vi "Emballage affiche cmde non terminée_V2.vi"(6 "error in (no error)":errorcluster caption="entrée d'erreur (pas d'erreur)", 11 "N° cmde en cours":string(combo)="02302/08-01.07.01", 16 "melange des lots possibles ?":bool=TRUE) -> (12 "DATA cmde":T1={"n°article FAS"="", "n° cmde FAS"="02302/08-01.07.01", "quantité cmde"="100", "ID LIG cmde"="225785", "n° cmde client"="120189 / 109644     ", "nom client"="Fluid Automat. Systems GmbH", "n° article client"="20869", "indice revision client"="03    ", "société de facturation"="FAS Medic SA                            ", "langue a utiliser"="ALL"}, 14 "Nombre de carton complets":i16=2, 15 "Nombre de carton+1 :":i16=2, 17 "pièce(s)":i16=8, 18 "#valve déjà emballée":i32, 19 "Commencer Une autre commande OUT":bool, 20 "Recommencer la commande OUT":bool, 21 "No commande FAS":string, 22 "Pb lecture cmde":bool, 23 "Continuer l'emballage  OUT":bool=TRUE, 24 "Quantité de la commande":string="4", 25 "Commande interne":bool, 26 "error out":errorcluster caption="sortie d'erreur")   [LabVIEW 2020]
uses:
  Modules/FS/60_FS_Controles/60_FS_SetGet.ctl
panel:
  out "temps [s]":dbl
  out "cmd non fini":string[](array[string])
  in  "Commencer Une autre commande":bool
  in  "Recommencer la commande":bool
  in  "Continuer l'emballage":bool
  # "Commande n°\n\nnon terminée !"
  # "Nombre de cartons emballés :"
  # "Vous avez \n dans le carton n°"
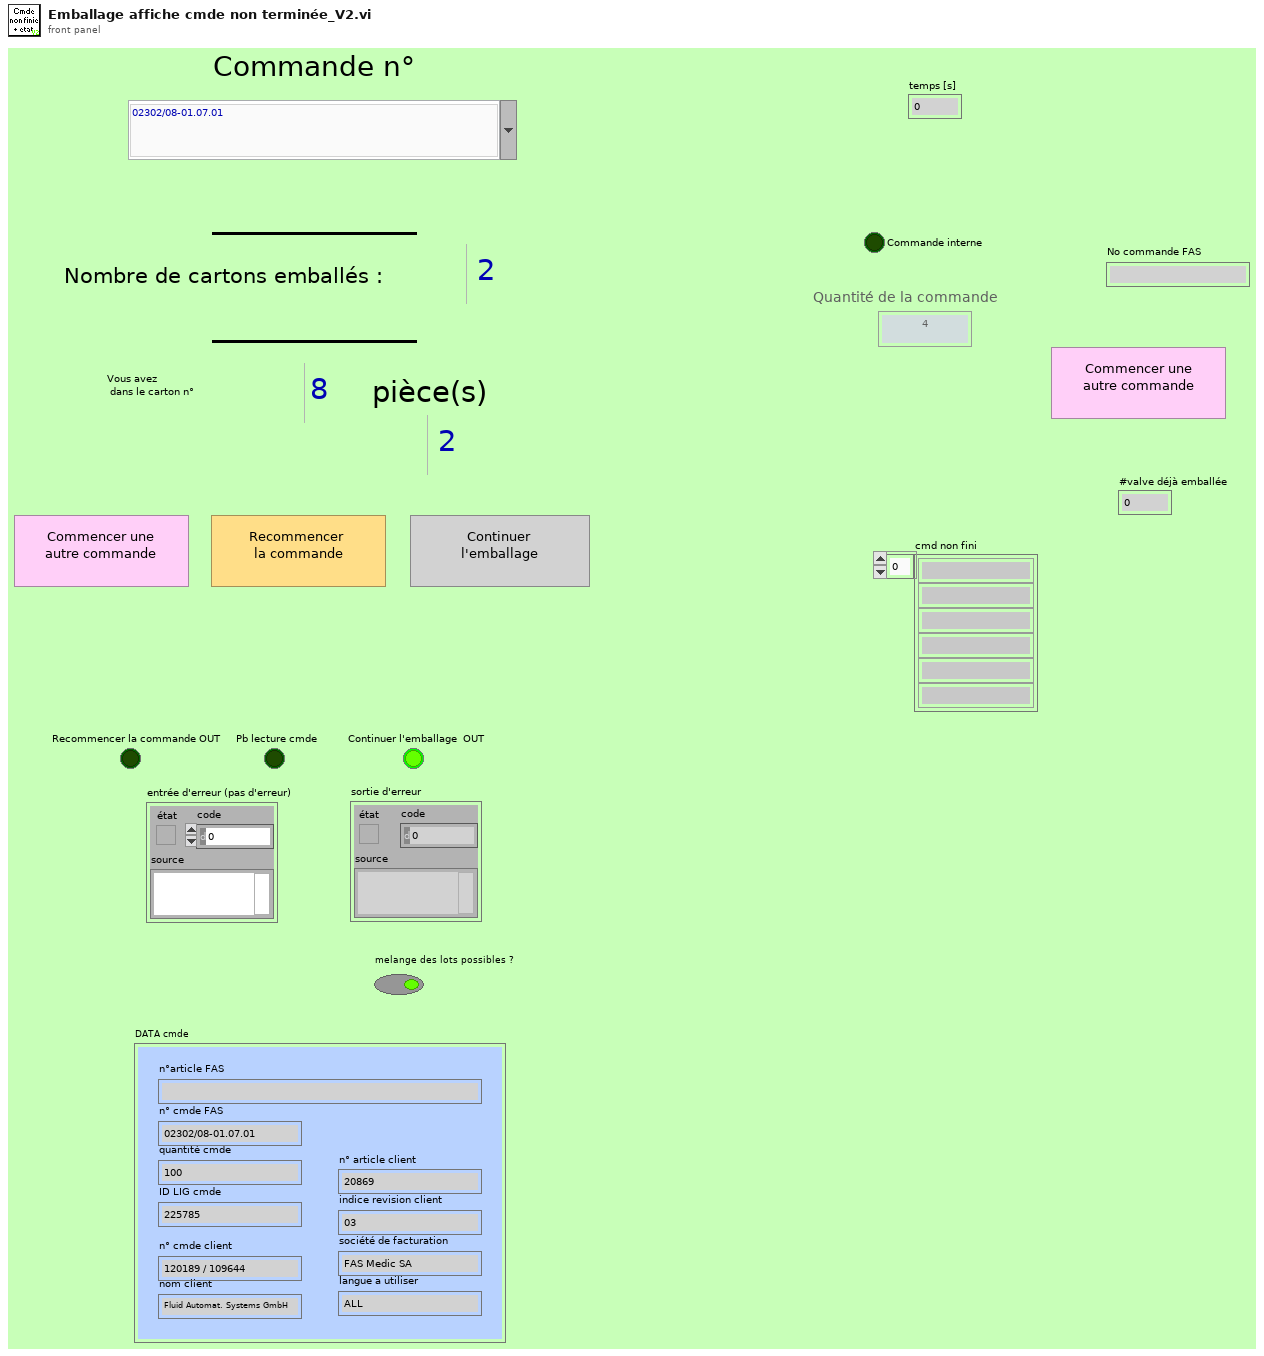
[diagram p1: front panel]
types:
  T1 = typedef "DATA commande.ctl" = cluster{"n°article FAS":string, "n° cmde FAS":string, "quantité cmde":string, "ID LIG cmde":string, "n° cmde client":string, "nom client":string, "n° article client":string, "indice revision client":string, "société de facturation":string, "langue a utiliser":string}
  T2 = enum8{"Enabled", "Disabled", "Disabled and Grayed Out"}
  T3 = typedef "60_FS_SetGet.ctl" = enum16{"set", "get"}
  T4 = typedef "Emballage_BDD_param_Produit.ctl" = cluster{"No_Valve_FAS":string, "suffixe":string, "designation":string, "indice_produit":string, "code_barre_fixe":string, "affiche_code_barre_client":string, "affiche_no_client":string, "Nb_vlve_par_carton":u16, "melange_des_lots_possible":string, "id_article":string, "Indice_Rev":string, "Famille":string, "date":string, "code_barre_fixe_Fin":string, "Longeur_No_Serie":string}
  T5 = typedef "60_FS_CLT_Chemins.ctl" = cluster{"Racine_local":path, "Racine_reseau":path, "Racine_Support_Application":path, "Fichier_Journalisation":path, "Connexion_BDD_VSX":path, "Connexion_BDD_PLZ":path}
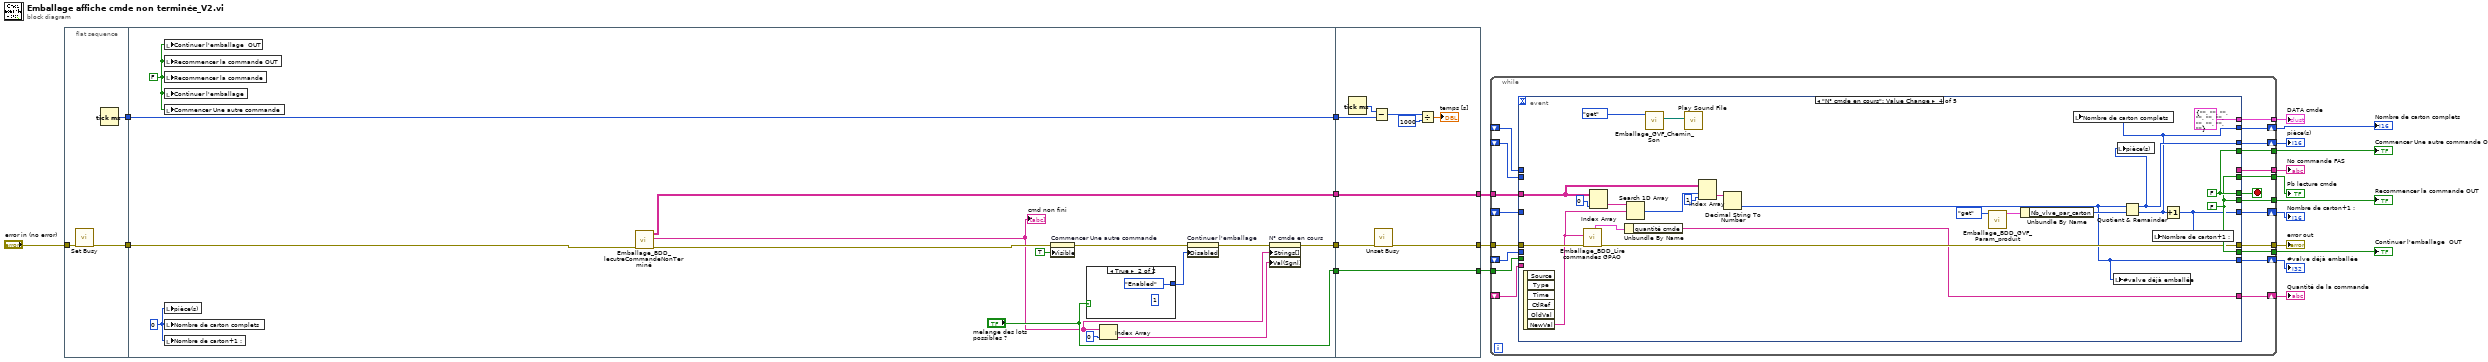
[diagram p0: block diagram]
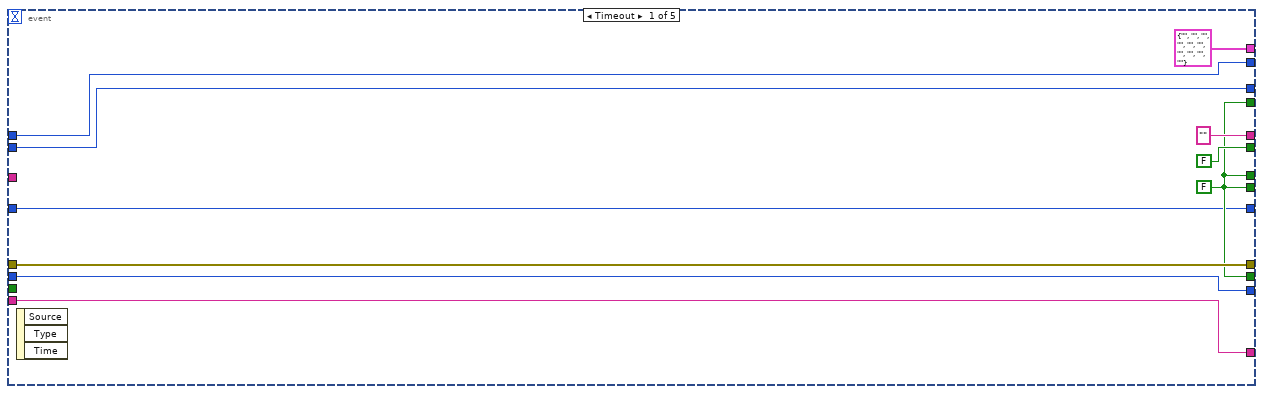
[diagram p2: hidden frame]
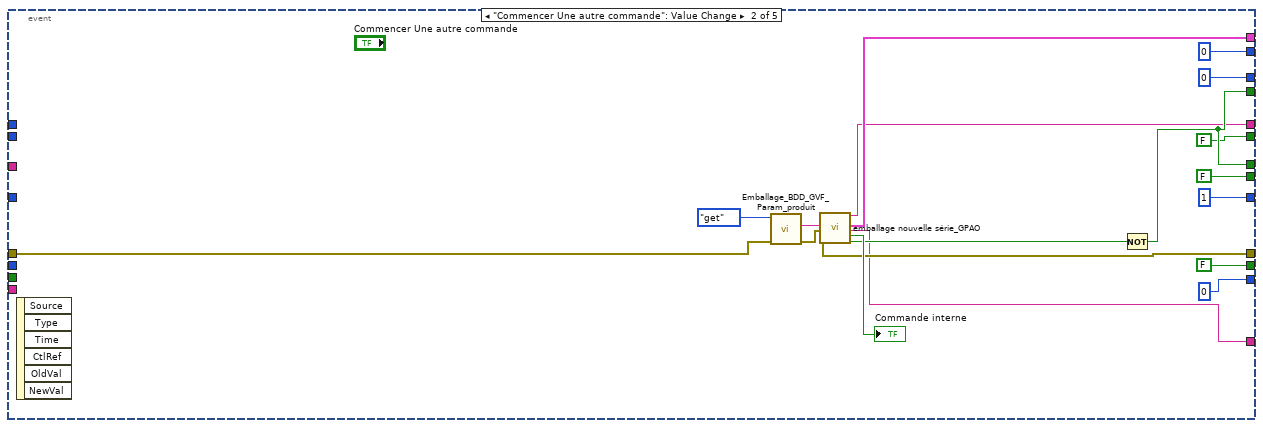
[diagram p3: hidden frame]
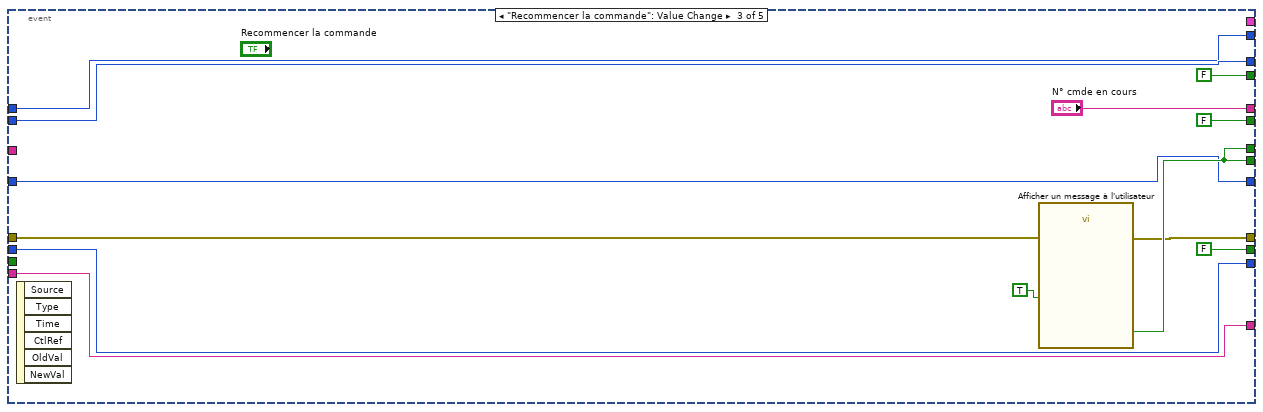
[diagram p4: hidden frame]
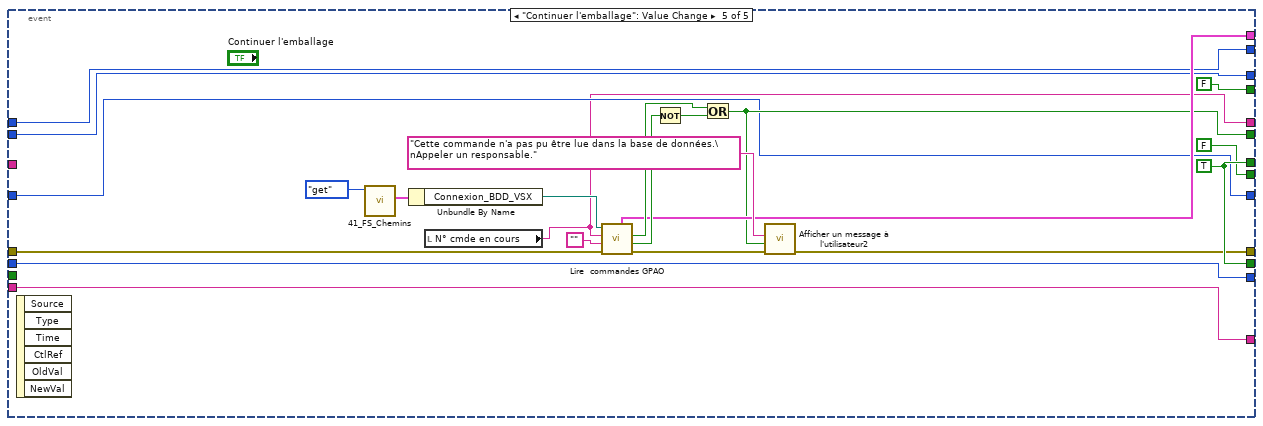
[diagram p5: hidden frame]
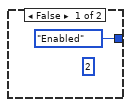
[diagram p6: hidden frame]
diagram:
  n1 = flat-sequence {
    tunnel: "error in (no error)" -> [w23]
    tunnel: [w24] -> w6
    tunnel: [w25] -> w2
    tunnel: w6 -> [w29]
    tunnel: [w35] -> w5
    tunnel: ["melange des lots possibles ?"] -> w4
    tunnel: [w26] -> w3
    tunnel: w2 -> [w30]
    tunnel: [w30] -> w1
    tunnel: [w49] -> w7
    tunnel: [w50] -> w13
    tunnel: [w43] -> w18
    tunnel: w5 -> [w51]
    tunnel: w4 -> [w50]
    tunnel: w3 -> [w49]
    tunnel: w1 -> [w47]
    frame #0 {
      n2 = call <vilib>:"Set Busy.vi"("error in (no error)"=w23) -> ("error out"=w24:errorcluster)  [unwired: 9 in, 1 out]
      n3 = Tick Count (ms)() -> (millisecond timer value=w25:u32)
    }
    frame #1 {
      w38 = i16 0 ("Nombre de carton+1 :")
      w39 = FALSE
      n4 = local write "Continuer l'emballage  OUT"(w39) -> ()
      n5 = local write "Recommencer la commande OUT"(w39) -> ()
      n6 = local write "Recommencer la commande"(w39) -> ()
      n7 = local write "Continuer l'emballage"(w39) -> ()
      n8 = local write "Commencer Une autre commande"(w39) -> ()
      n9 = local write "pièce(s)"(w38) -> ()
      n10 = local write "Nombre de carton complets"(w38) -> ()
      n11 = local write "Nombre de carton+1 :"(w38) -> ()
      n12 = call "Emballage_BDD_lecutreCommandeNonTerminé.vi"("entrée d'erreur (pas d'erreur)"=w29) -> ("sortie d'erreur"=w28:errorcluster, "Cmd_nonFini"=w27:string[], "Liste des champs à lire 2"=w26:string[][])  [unwired: 8 in]
      "cmd non fini" <- w27
      n13 = property on="Commencer Une autre commande" class="Bool (strict)"(error in=w28, "Visible"=TRUE) -> (error out=w32:errorcluster)  [unwired: 1 in, 1 out]
      n14 = case shown="True" "melange des lots possibles ?" {
        tunnel: [T2."Enabled" ("Désactivé") T2."Enabled" ("Désactivé")] -> w40
        frame False {
          (unwired) 2
        }
        frame True {
          (unwired) 1
        }
      }
      n15 = Index Array(array=w27, index=0 ("indice")) -> (element=w31:string)
      n16 = property on="Continuer l'emballage" class="Bool (strict)"(error in=w32, "Disabled"=w40) -> (error out=w36:errorcluster)  [unwired: 1 in, 1 out]
      n17 = property on="N° cmde en cours" class="CmbBox"(error in=w36, "Strings[]"=w27, "Val(Sgnl)"=w31) -> (error out=w35:errorcluster)  [unwired: 1 in, 1 out]
    }
    frame #2 {
      n18 = Tick Count (ms)() -> (millisecond timer value=w48:u32)
      n19 = Subtract(x=w48, y=w47) -> (x-y=w46:u32)
      n20 = call <vilib>:"Unset Busy.vi"("error in (no error)"=w51) -> ("error out"=w43:errorcluster)  [unwired: 10 in]
      n21 = Divide(x=w46, y=u32 1000) -> (x/y=→"temps [s]":dbl)
    }
  }
  n22 = while {
    tunnel: [w71] -> w21
    tunnel: [w70] -> w20
    tunnel: [w69] -> w19
    tunnel: [w68] -> w15
    tunnel: [w67] -> w14
    tunnel: w18 -> [w66]
    tunnel: [w65] -> w17
    tunnel: [w64] -> w16
    tunnel: w13 -> [w63]
    shift-right: [w62] -> w12
    shift-left: _ -> [w57]
    shift-right: [w61] -> w11
    shift-left: _ -> [w58]
    shift-right: [w60] -> w10
    shift-left: _ -> [w59]
    shift-right: [w56] -> w9
    shift-left: _ -> [w53]
    shift-right: [w55] -> w8
    shift-left: _ -> [w54]
    tunnel: w7 -> [w52]
    stop <- w72 stop-if-true
    n23 = event shown="[3] \"N° cmde en cours\": Value Change" {
      selector: _ -> [_ _ _ _ _]
      dyn-events: _ -> [_ _ _ _ _]
      timeout: _ -> [_ _ _ _ _]
      tunnel: [w78 w99 w112 w136 w158] -> w72
      tunnel: [w78 w99 FALSE w136 FALSE] -> w71
      tunnel: [w78 FALSE ("OK") w112 w134 FALSE ("OK")] -> w70
      tunnel: [w78 FALSE ("OK") FALSE ("OK") w134 w158] -> w69
      tunnel: [T1 {"n°article FAS"="", "n° cmde FAS"="", "quantité cmde"="", "ID LIG cmde"="", "n° cmde client"="", "nom client"="", "n° article client"="", "indice revision client"="", "société de facturation"="", "langue a utiliser"=""} ("DATA cmde") w95 _ T1 {"n°article FAS"="", "n° cmde FAS"="", "quantité cmde"="", "ID LIG cmde"="", "n° cmde client"="", "nom client"="", "n° article client"="", "indice revision client"="", "société de facturation"="", "langue a utiliser"=""} ("DATA cmde") w151] -> w68
      tunnel: [w82 w98 w110 w128 w150] -> w67
      tunnel: w66 -> [w82 w84 w111 w130 w149]
      tunnel: ["" ("N° cmde en cours") w94 "N° cmde en cours" _ w137] -> w65
      tunnel: [FALSE FALSE FALSE w134 w148] -> w64
      tunnel: w63 -> [_ _ _ _ _]
      tunnel: [w77 0 w103 w118 w140] -> w62
      tunnel: [w76 1 w104 w117 w141] -> w61
      tunnel: [w75 0 w105 w119 w142] -> w60
      tunnel: w59 -> [w75 _ w105 _ w142]
      tunnel: w58 -> [w76 _ w104 _ w141]
      tunnel: w57 -> [w77 _ w103 _ w140]
      tunnel: [w74 0 w106 w116 w139] -> w56
      tunnel: w53 -> [w74 _ w106 _ w139]
      tunnel: [w73 w87 w102 w127 w138] -> w55
      tunnel: w54 -> [w73 _ w102 _ w138]
      tunnel: w52 -> [_ _ _ w122 _]
      event Timeout {
        w78 = FALSE
        n24 = event-data() -> ()  [unwired: 1 in, 3 out]
      }
      event "Commencer Une autre commande": Value Change {
        n25 = event-data() -> ()  [unwired: 1 in, 6 out]
        n26 = call "Emballage_BDD_GVF_Param_produit.vi"("Error in"=w84, "Énum"=enum16{"set", "get"}."get") -> ("Error out"=w83:errorcluster, "Produit OUT"=w85:string)  [unwired: 6 in, 2 out]
        n27 = call "emballage nouvelle série_GPAO.vi"("Nom du produit"=w85, "error in (no error)"=w83) -> ("error out"=w98:errorcluster, "No commande FAS"=w94:string, "DATA cmde"=w95:T1, "Quantité de la commande"=w87:string, "Commande interne"=→"Commande interne":bool, "Annuler(T=OK)"=w97:bool)  [unwired: 11 in, 1 out]
        n28 = Not(x=w97) -> (.not. x?=w99:bool)
      }
      event "Recommencer la commande": Value Change {
        n29 = event-data() -> ()  [unwired: 1 in, 6 out]
        n30 = call "Afficher un message à l'utilisateur"("error in (no error)"=w111, "Enable"=TRUE) -> ("error out"=w110:errorcluster, "OK"=w112:bool)  [unwired: 8 in]
      }
      event "N° cmde en cours": Value Change {
        w134 = FALSE ("OK")
        w136 = FALSE ("OK")
        n31 = event-data() -> ("NewVal"=w124:string)  [unwired: 1 in, 5 out]
        n32 = call "Emballage_BDD_Lire  commandes GPAO.vi"("error in"=w130, "Numéro commande"=w124) -> ("error out"=w128:errorcluster, "DATA cmde"=w131:T1)  [unwired: 4 in, 4 out]
        n33 = Index Array(array=w122, index (col)=0 ("indice désactivé (col)")) -> (element=w125:string[])  [unwired: 1 in]
        n34 = Unbundle By Name(w131) -> ("quantité cmde"=w127:string)
        n35 = Search 1D Array(1D array=w125, element=w124) -> (index of element=w121:i32)  [unwired: 1 in]
        n36 = call "Emballage_GVF_Chemin_Son.vi"("Énum"=enum16{"get", "set"}."get") -> ("Chemin Utopia - Question.WAV"=w132:path)  [unwired: 6 in, 4 out]
        n37 = call <vilib>:"Play Sound File.vi"("path"=w132) -> ()  [unwired: 9 in, 2 out]
        n38 = Index Array(array=w122, index (row)=w121, index (col)=1 ("indice désactivé (col)")) -> (element=w120:string)
        n39 = Decimal String To Number(string=w120) -> (number=w116:i32)  [unwired: 2 in, 1 out]
        n40 = call "Emballage_BDD_GVF_Param_produit.vi"("Énum"=enum16{"set", "get"}."get") -> ("CLS_param_produit"=w115:T4)  [unwired: 7 in, 3 out]
        n41 = Unbundle By Name(w115) -> ("Nb_vlve_par_carton"=w129:u16)
        n42 = local write "#valve déjà emballée"(w116) -> ()
        n43 = Quotient & Remainder(x=w116, y=w129) -> (x-y*floor(x/y)=w119:i32, floor(x/y)=w118:i32)
        n44 = local write "Nombre de carton complets"(w118) -> ()
        n45 = local write "pièce(s)"(w119) -> ()
        n46 = Increment(x=w118) -> (x+1=w117:i32)
        n47 = local write "Nombre de carton+1 :"(w117) -> ()
      }
      event "Continuer l'emballage": Value Change {
        w158 = TRUE ("OK")
        n48 = event-data() -> ()  [unwired: 1 in, 6 out]
        n49 = call "41_FS_Chemins.vi"("SetGet"=60_FS_SetGet."get") -> ("CLT_Chemins_out"=w145:T5)  [unwired: 9 in, 1 out]
        n50 = Unbundle By Name(w145) -> ("Connexion_BDD_VSX"=w143:path)
        n51 = local read "N° cmde en cours"() -> (w137:string)
        n52 = call "Lire  commandes GPAO.vi"("error in"=w149, "article"="", "Numéro commande"=w137, "connection information"=w143) -> ("error out"=w155:errorcluster, "existe ?"=w157:bool, "Erreur de\n comunication"=w156:bool, "DATA cmde"=w151:T1)  [unwired: 3 in, 1 out]
        n53 = Not(x=w157) -> (.not. x?=w154:bool)
        n54 = Or(x=w156, y=w154) -> (x .or. y?=w148:bool)
        n55 = call "Afficher un message à l'utilisateur2"("error in (no error)"=w155, "Enable"=w148, "Message"="Cette commande n'a pas pu être lue dans la base de données.\nAppeler un responsable.") -> ("error out"=w150:errorcluster)  [unwired: 7 in, 1 out]
      }
    }
  }
  "error out" <- w14
  "No commande FAS" <- w17
  "DATA cmde" <- w15
  "Commencer Une autre commande OUT" <- w21
  "Recommencer la commande OUT" <- w20
  "Continuer l'emballage  OUT" <- w19
  "Pb lecture cmde" <- w16
  "Nombre de carton complets" <- w12
  "Nombre de carton+1 :" <- w11
  "pièce(s)" <- w10
  "#valve déjà emballée" <- w9
  "Quantité de la commande" <- w8
